vi "Database Settings Window.vi"() -> ()   [LabVIEW 2019]
uses:
  <vilib>/Utility/config.llb/Write Key (String).vi
  <vilib>/Utility/config.llb/NI_LVConfig.lvlib
panel:
  in  "Database Connection":T1={"Data Source Name"="HANSPH_LAPTOP\\SQLEXPRESS", "Database Name"="MEASUREMENTS", "User Name"="sa", "Password"="Ullabella72"}
  in  "Cancel Button":bool
  in  "OK Button":bool
  out "Error Out":errorcluster
  in  "Error In":errorcluster
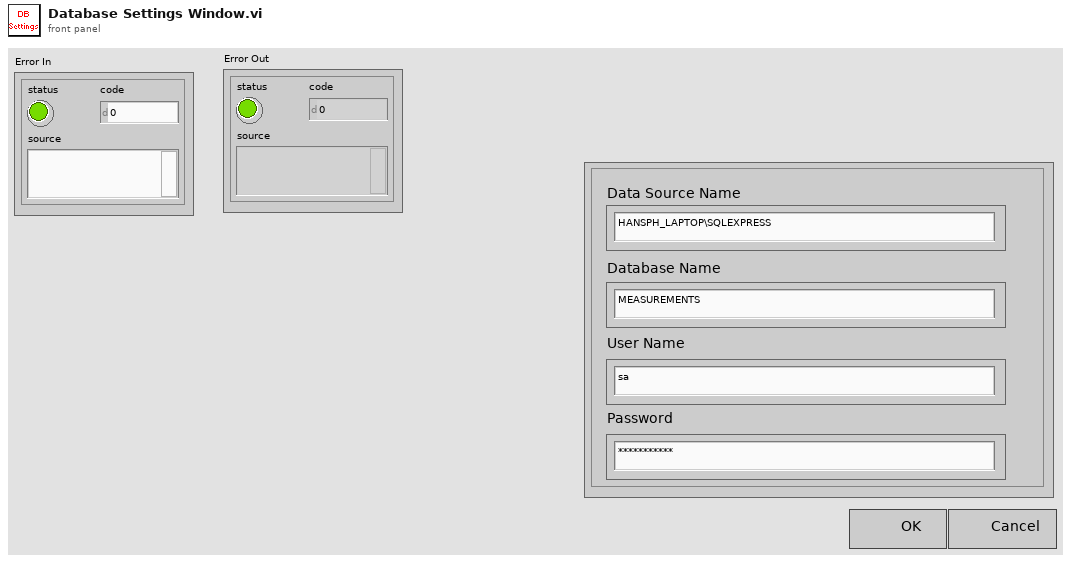
[diagram p1: front panel]
types:
  T1 = cluster{"Data Source Name":string, "Database Name":string, "User Name":string, "Password":string}
  T2 = typedef "NI_LVConfig.lvlib/Config Data RefNum.ctl" = refnum<k1>
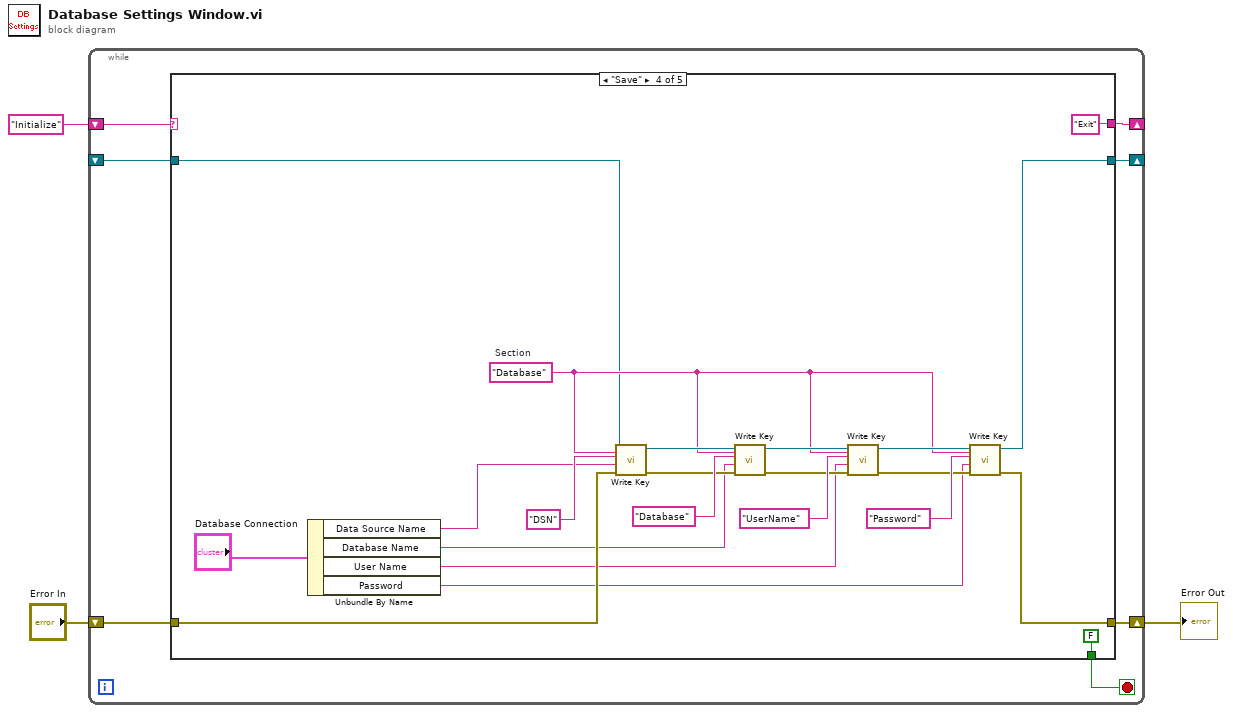
[diagram p0: block diagram]
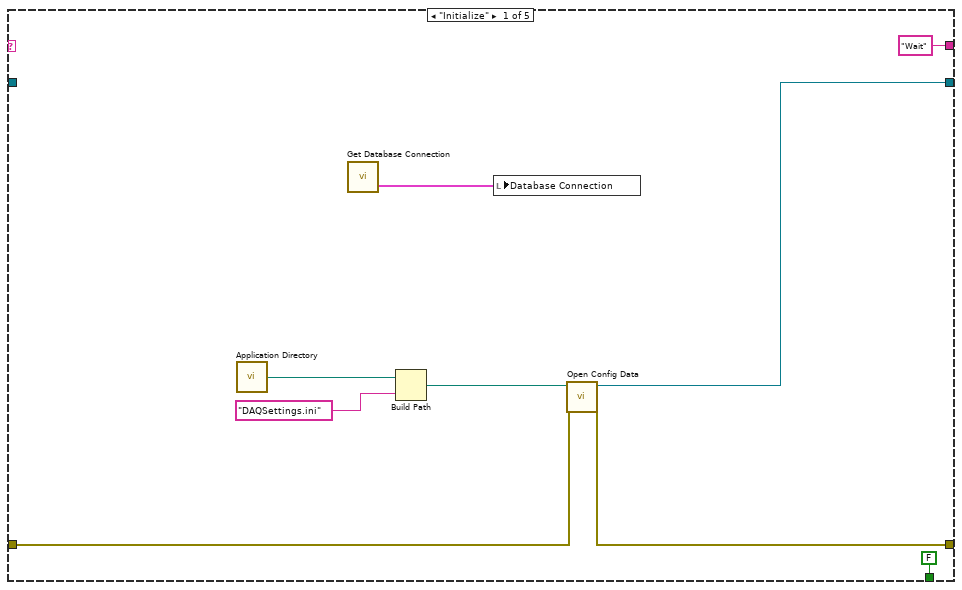
[diagram p2: hidden frame]
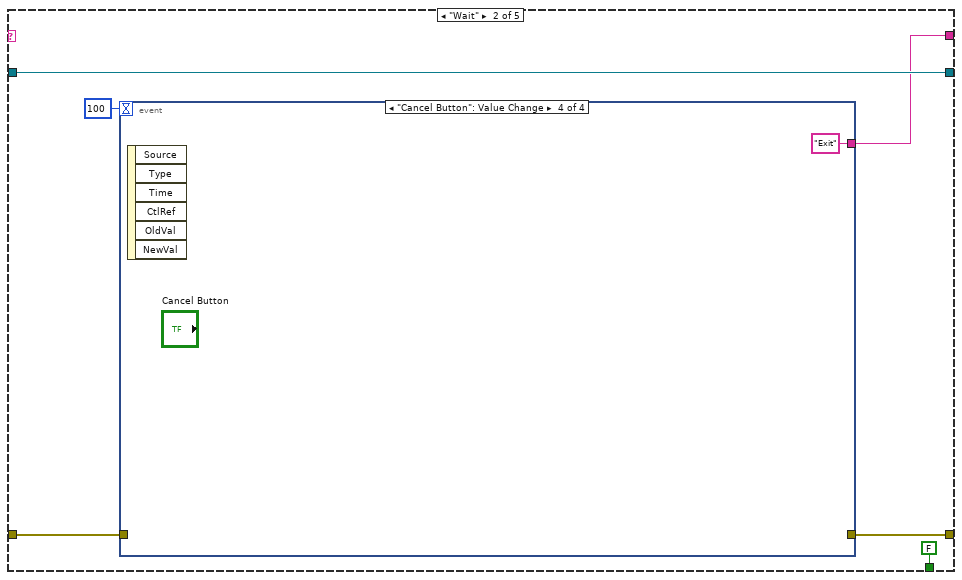
[diagram p3: hidden frame]
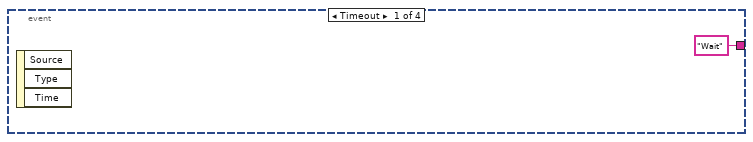
[diagram p4: hidden frame]
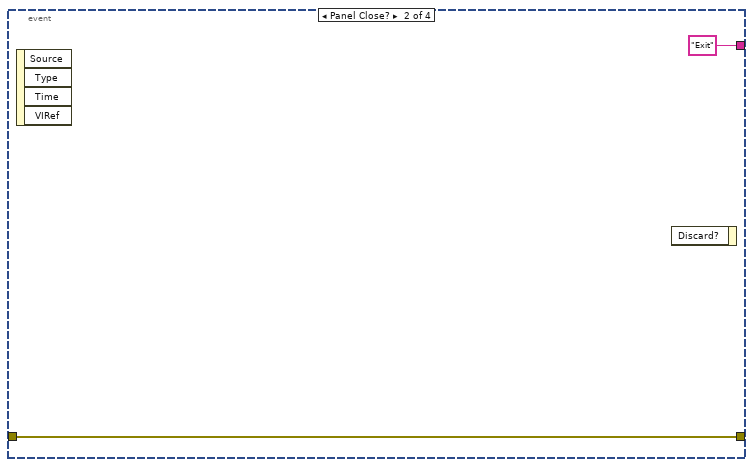
[diagram p5: hidden frame]
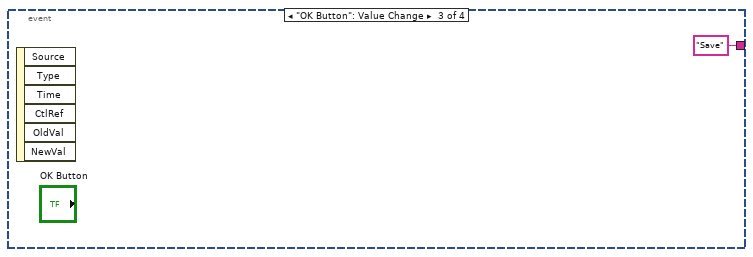
[diagram p6: hidden frame]
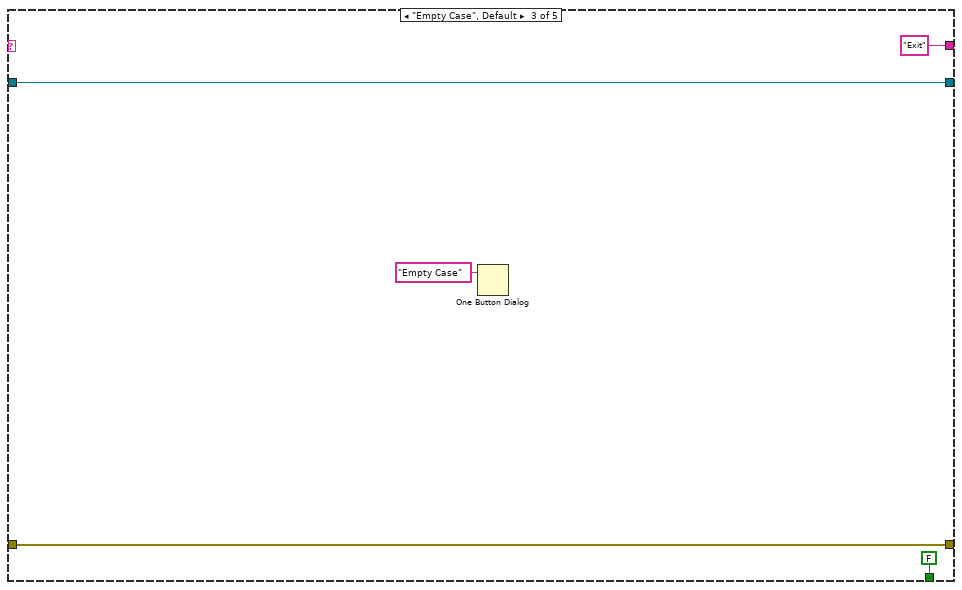
[diagram p7: hidden frame]
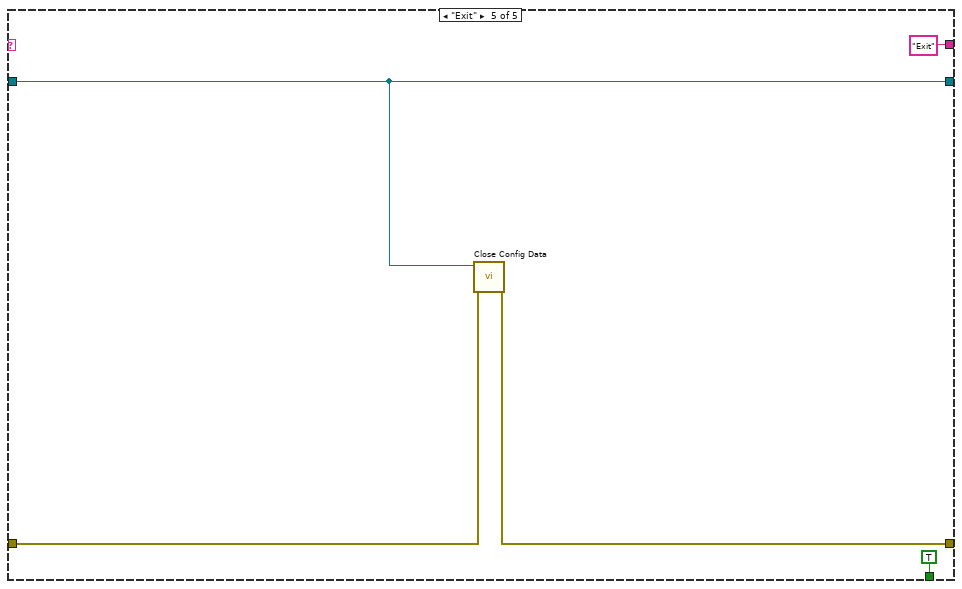
[diagram p8: hidden frame]
diagram:
  n1 = while {
    shift-right: [w6] -> _
    shift-left: "Initialize" ("key") -> [w10]
    shift-right: [w7] -> _
    shift-left: _ -> [w9]
    shift-right: [w4] -> w1
    shift-left: "Error In" -> [w8]
    stop <- w5 stop-if-true
    n2 = case shown="\"Save\"" w10 {
      tunnel: w9 -> [_ w24 w32 w41 w60]
      tunnel: w8 -> [w12 w21 w33 w43 w59]
      tunnel: [w13 w24 w32 w40 w60] -> w7
      tunnel: ["Wait" ("key") w23 "Exit" ("key") "Exit" ("key") "Exit" ("key")] -> w6
      tunnel: [FALSE FALSE FALSE FALSE TRUE] -> w5
      tunnel: [w11 w20 w33 w42 w58] -> w4
      frame "Initialize" {
        n3 = call <vilib>:"Application Directory.vi"() -> ("Application Directory"=w16:path)
        n4 = call "Get Database Connection.vi"() -> ("Database Settings"=w17:T1)  [unwired: 2 in, 1 out]
        n5 = Build Path(base path=w16, name or relative path="DAQSettings.ini") -> (appended path=w14:path)
        n6 = local write "Database Connection"(w17) -> ()
        n7 = call <vilib>:"Open Config Data.vi"("error in (no error)"=w12, "configuration file path"=w14) -> ("error out"=w11:errorcluster, "refnum"=w13:T2)  [unwired: 7 in, 1 out]
      }
      frame "Wait" {
        n8 = event shown="[3] \"Cancel Button\": Value Change" {
          selector: _ -> [_ _ _ _]
          dyn-events: _ -> [_ _ _ _]
          timeout: 100 -> [_ _ _ _]
          tunnel: ["Wait" ("key") "Exit" ("key") "Save" ("key") "Exit" ("key")] -> w23
          tunnel: w21 -> [_ w27 _ _]
          tunnel: [_ w27 _ _] -> w20
          event Timeout {
            n9 = event-data() -> ()  [unwired: 1 in, 3 out]
          }
          event Panel Close? {
            n10 = event-data() -> ()  [unwired: 1 in, 4 out]
            n11 = event-data() -> ()  [unwired: 2 in, 1 out]
          }
          event "OK Button": Value Change {
            n12 = event-data() -> ()  [unwired: 1 in, 6 out]
          }
          event "Cancel Button": Value Change {
            n13 = event-data() -> ()  [unwired: 1 in, 6 out]
          }
        }
      }
      frame "Empty Case", Default {
        n14 = One Button Dialog(message="Empty Case") -> ()  [unwired: 1 in, 1 out]
      }
      frame "Save" {
        w45 = "Database"  # Section
        n15 = Unbundle By Name("Database Connection") -> ("Data Source Name"=w39:string, "Database Name"=w38:string, "User Name"=w37:string, "Password"=w36:string)
        n16 = call-poly <vilib>:"Write Key.vi"("section"=w45, "error in (no error)"=w43, "value"=w39, "key"="DSN", "refnum"=w41) -> ("error out"=w54:errorcluster, "refnum out"=w53:T2)  [unwired: 4 in, 1 out]
        n17 = call-poly <vilib>:"Write Key.vi"("section"=w45, "error in (no error)"=w54, "value"=w38, "key"="Database", "refnum"=w53) -> ("error out"=w48:errorcluster, "refnum out"=w49:T2)  [unwired: 4 in, 1 out]
        n18 = call-poly <vilib>:"Write Key.vi"("section"=w45, "error in (no error)"=w48, "value"=w37, "key"="UserName", "refnum"=w49) -> ("error out"=w46:errorcluster, "refnum out"=w47:T2)  [unwired: 4 in, 1 out]
        n19 = call-poly <vilib>:"Write Key.vi"("section"=w45, "error in (no error)"=w46, "value"=w36, "key"="Password", "refnum"=w47) -> ("error out"=w42:errorcluster, "refnum out"=w40:T2)  [unwired: 4 in, 1 out]
      }
      frame "Exit" {
        n20 = call <vilib>:"Close Config Data.vi"("error in (no error)"=w59, "refnum"=w60) -> ("error out"=w58:errorcluster)  [unwired: 8 in, 1 out]
      }
    }
  }
  "Error Out" <- w1
